vi "Get All Channel Refs.vi"(8 "error in (no error)":errorcluster, 10 "framework configuration in":T1, 11 "VeriStand Data Sharing Framework in":refnum<class "VeriStand DSF.lvclass">) -> (0 "error out":errorcluster, 1 "contiguous?":bool, 2 "all channel offsets":u64[](array[numeric]) format="%.0x", 3 "VeriStand Data Sharing Framework out":refnum<class "VeriStand DSF.lvclass">)   [LabVIEW 2017, in "DSF Engine.lvlib" / "VeriStand DSF.lvclass"]
uses:
  VeriStand DSF.lvclass
  DSF Core.lvlibp/Typedefs/DSF Engine Framework Configuration.ctl
  DSF Core.lvlibp/Typedefs/DSF Engine Plugin Configuration.ctl
  DSF Core.lvlibp/Typedefs/DSF Timing Info.ctl
  DSF Core.lvlibp/Typedefs/DSF Engine Plugin Thread Configuration.ctl
  DSF Core.lvlibp/Typedefs/DSF Settings Info.ctl
  DSF Core.lvlibp/Typedefs/DSF Engine Transfer Group Configuration.ctl
  DSF Core.lvlibp/Typedefs/DSF Direction.ctl
  DSF Core.lvlibp/Typedefs/DSF Engine Transfer Configuration.ctl
  DSF Core.lvlibp/Typedefs/DSF Byte Order.ctl
  DSF Core.lvlibp/Typedefs/DSF Engine Channel Configuration.ctl
  DSF Core.lvlibp/Typedefs/DSF Data Type.ctl
  DSF Core.lvlibp/Typedefs/DSF Timeout Behavior.ctl
  VeriStand DSF.lvclass/VeriStand DSF.ctl
  <vilib>/NI Veristand/Custom Device API/Data Access Type.ctl
  DSF Core.lvlibp/Classes/Configuration/Channel Count (Transfer).vi
  <vilib>/NI Veristand/Custom Device API/Custom Device API.lvlib
  DSF Core.lvlibp
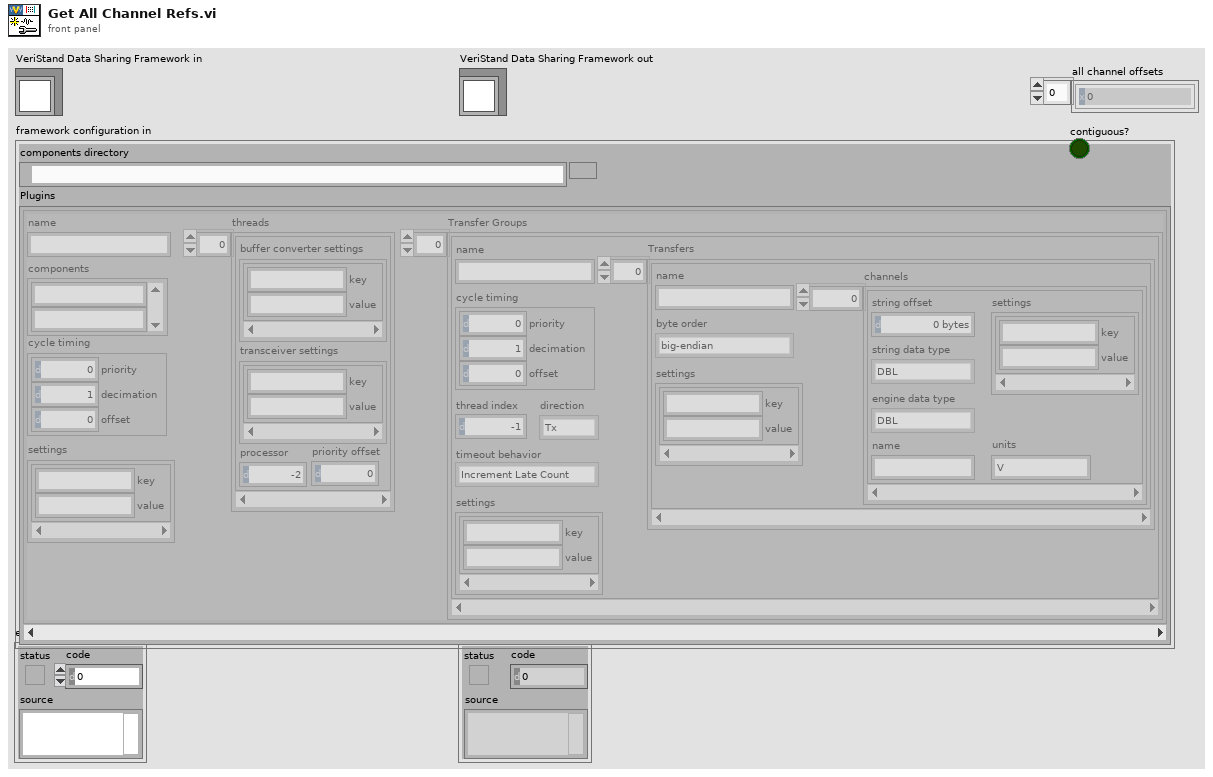
[diagram p1: front panel]
types:
  T1 = typedef "DSF Core.lvlibp/DSF Engine Framework Configuration.ctl" = cluster{"components directory":path, "Plugins":T2[]}
  T2 = typedef "DSF Core.lvlibp/DSF Engine Plugin Configuration.ctl" = cluster{"name":string, "components":string[], "cycle timing":T3, "threads":T4[], "Transfer Groups":T6[], "settings":T5}
  T3 = typedef "DSF Core.lvlibp/DSF Timing Info.ctl" = cluster{"priority":u64, "decimation":u64, "offset":u64}
  T4 = typedef "DSF Core.lvlibp/DSF Engine Plugin Thread Configuration.ctl" = cluster{"buffer converter settings":T5, "transceiver settings":T5, "processor":i32, "priority offset":i16}
  T5 = typedef "DSF Core.lvlibp/DSF Settings Info.ctl" = cluster{"key":string, "value":string}[]
  T6 = typedef "DSF Core.lvlibp/DSF Engine Transfer Group Configuration.ctl" = cluster{"name":string, "direction":T7, "cycle timing":T3, "thread index":i32, "settings":T5, "Transfers":T8[], "timeout behavior":T12}
  T7 = typedef "DSF Core.lvlibp/DSF Direction.ctl" = enum8{"Tx", "Rx"}
  T8 = typedef "DSF Core.lvlibp/DSF Engine Transfer Configuration.ctl" = cluster{"name":string, "byte order":T9, "settings":T5, "channels":T10[]}
  T9 = typedef "DSF Core.lvlibp/DSF Byte Order.ctl" = enum8{"big-endian", "little-endian"}
  T10 = typedef "DSF Core.lvlibp/DSF Engine Channel Configuration.ctl" = cluster{"string offset":u64, "string data type":T11, "engine data type":T11, "name":string, "settings":T5, "units":string}
  T11 = typedef "DSF Core.lvlibp/DSF Data Type.ctl" = enum8{"Bool", "SGL", "DBL", "I8", "I16", "I32", "I64", "U8", "U16", "U32", "U64"}
  T12 = typedef "DSF Core.lvlibp/DSF Timeout Behavior.ctl" = enum8{"Increment Late Count", "Throw Error"}
  T13 = enum16{"open", "replace", "create", "open or create", "replace or create", "replace or create with confirmation"}
  T14 = typedef "Custom Device API.lvlib/Custom Device Item Ref.ctl" = u64
  T15 = typedef "Custom Device API.lvlib/Data Access Type.ctl" = enum16{"Read", "Write"}
  T16 = typedef "Custom Device API.lvlib/Data Reference.ctl" = i32
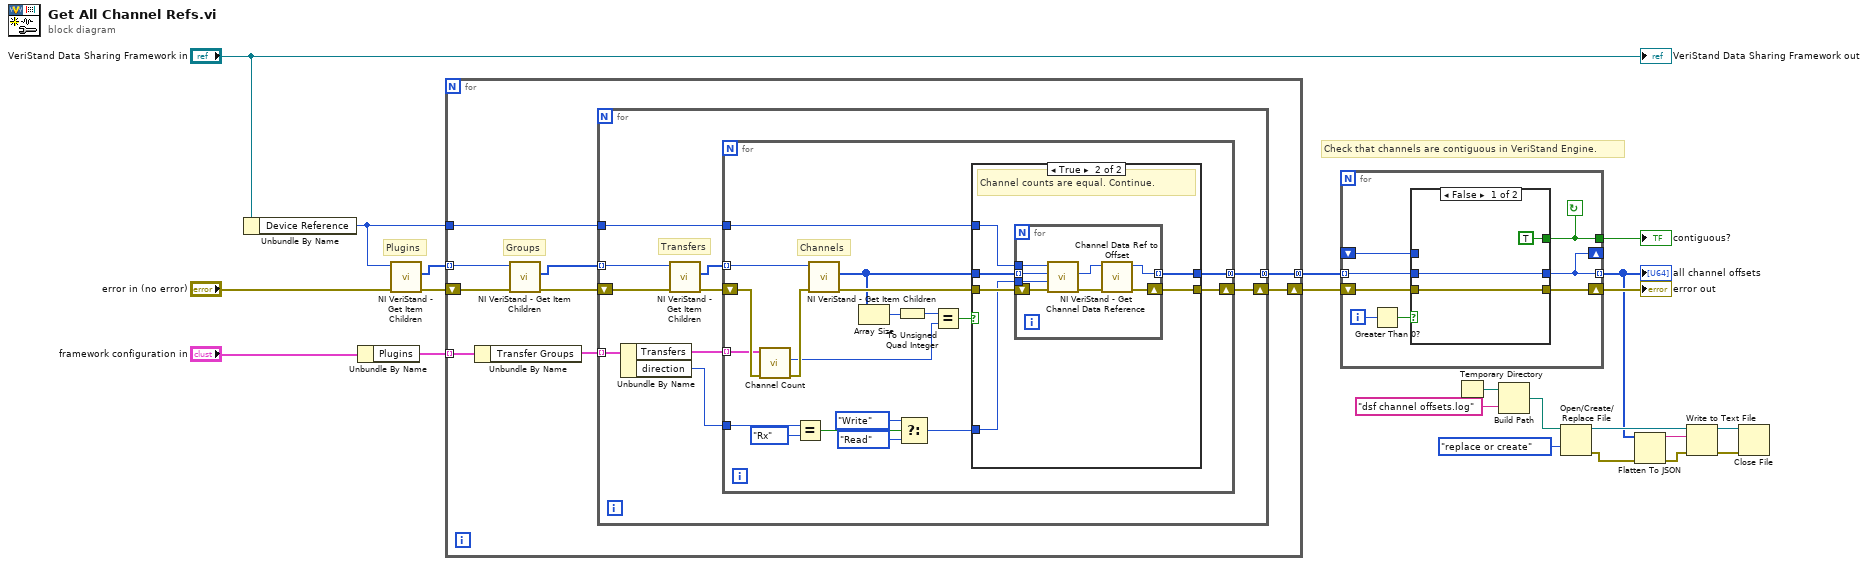
[diagram p0: block diagram]
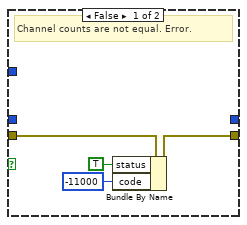
[diagram p2: hidden frame]
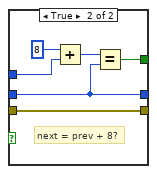
[diagram p3: hidden frame]
diagram:
  # "Check that channels are contiguous in VeriStand Engine."
  # "Plugins"
  n1 = Unbundle By Name("VeriStand Data Sharing Framework in") -> ("Device Reference"=w18:T14)
  n2 = Unbundle By Name("framework configuration in") -> ("Plugins"=w19:T2[])
  n3 = call <vilib>:"NI VeriStand - Get Item Children.vi"("error in (no error)"="error in (no error)", "Item Ref in"=w18) -> ("error out"=w17:errorcluster, "Child Refs"=w20:T14[])  [unwired: 6 in, 2 out]
  n4 = for {
    tunnel: w20 -> [w30] mode=indexing
    tunnel: w19 -> [w31] mode=indexing
    tunnel: w18 -> [w29]
    shift-right: [w27] -> w15
    shift-left: w17 -> [w28]
    tunnel: [w26] -> w14 mode=concatenating
    # "Groups"
    n5 = Unbundle By Name(w31) -> ("Transfer Groups"=w25:T6[])
    n6 = call <vilib>:"NI VeriStand - Get Item Children.vi"("error in (no error)"=w28, "Item Ref in"=w30) -> ("error out"=w23:errorcluster, "Child Refs"=w24:T14[])  [unwired: 6 in, 2 out]
    n7 = for {
      tunnel: w25 -> [w40] mode=indexing
      tunnel: w24 -> [w41] mode=indexing
      tunnel: w29 -> [w39]
      shift-right: [w37] -> w27
      shift-left: w23 -> [w38]
      tunnel: [w36] -> w26 mode=concatenating
      # "Transfers"
      n8 = Unbundle By Name(w40) -> ("Transfers"=w35:T8[], "direction"=w32:T7)
      n9 = call <vilib>:"NI VeriStand - Get Item Children.vi"("error in (no error)"=w38, "Item Ref in"=w41) -> ("error out"=w33:errorcluster, "Child Refs"=w34:T14[])  [unwired: 6 in, 2 out]
      n10 = for {
        tunnel: w35 -> [w44] mode=indexing
        tunnel: w34 -> [w60] mode=indexing
        tunnel: w32 -> [w58]
        tunnel: w39 -> [w51]
        shift-right: [w43] -> w37
        shift-left: w33 -> [w47]
        tunnel: [w42] -> w36 mode=concatenating
        # "Channels"
        n11 = call-poly "Channel Count.vi"("error in (no error)"=w47, "Transfer Configuration in"=w44) -> ("error out"=w46:errorcluster, "total channel count"=w45:u64)  [unwired: 7 in, 1 out]
        n12 = Equal?(x=w58, y=DSF_Direction."Rx") -> (x = y?=w56:bool)
        n13 = call <vilib>:"NI VeriStand - Get Item Children.vi"("error in (no error)"=w46, "Item Ref in"=w60) -> ("error out"=w49:errorcluster, "Child Refs"=w48:T14[])  [unwired: 6 in, 2 out]
        n14 = Array Size(array=w48) -> (size(s)=w59:i32)
        n15 = To Unsigned Quad Integer(1:w59) -> (0:w52:u64)
        n16 = Select(t=Data_Access_Type."Write" ("Access"), s=w56, f=Data_Access_Type."Read") -> (s? t:f=w50:T15)
        n17 = Equal?(x=w52, y=w45) -> (x = y?=w53:bool)
        n18 = case shown="True" w53 {
          tunnel: w48 -> [_ w67]
          tunnel: w51 -> [_ w69]
          tunnel: w50 -> [_ w68]
          tunnel: w49 -> [w64 w70]
          tunnel: [w63 w65] -> w43
          tunnel: [_ w66] -> w42
          frame False {
            # "Channel counts are not equal. Error."
            n19 = Bundle By Name(cluster=w64, "status"=TRUE, "code"=-11000) -> (w63:errorcluster)
          }
          frame True {
            # "Channel counts are equal. Continue."
            n20 = for {
              tunnel: w69 -> [w77]
              tunnel: w68 -> [w76]
              tunnel: w67 -> [w75] mode=indexing
              tunnel: [w71] -> w66 mode=indexing
              shift-right: [w72] -> w65
              shift-left: w70 -> [w78]
              n21 = call <vilib>:"NI VeriStand - Get Channel Data Reference.vi"("error in (no error)"=w78, "Access"=w76, "Channel Ref in"=w75, "Device Ref in"=w77) -> ("error out"=w74:errorcluster, "Channel Data Reference"=w73:T16)  [unwired: 5 in, 1 out]
              n22 = call "Channel Data Ref to Offset.vi"("error in (no error)"=w74, "Channel Data Reference"=w73) -> ("error out"=w72:errorcluster, "channel offset"=w71:u64)  [unwired: 8 in]
            }
          }
        }
      }
    }
  }
  n23 = for {
    tunnel: w14 -> [w84] mode=indexing
    shift-right: [w81] -> w13
    shift-left: w15 -> [w83]
    shift-right: [w79] -> _
    shift-left: _ -> [w82]
    tunnel: [w80] -> w12
    tunnel: [w79] -> w1 mode=indexing
    i -> [w86]
    stop <- w80 continue-if-true
    n24 = Greater Than 0?(x=w86) -> (x > 0?=w85:bool)
    n25 = case shown="False" w85 {
      tunnel: w84 -> [w88 w91]
      tunnel: w83 -> [w89 w90]
      tunnel: w82 -> [_ w95]
      tunnel: [w89 w90] -> w81
      tunnel: [TRUE w92] -> w80
      tunnel: [w88 w91] -> w79
      frame False {
      }
      frame True {
        # "next = prev + 8?"
        n26 = Add(x=u64 8 ("y"), y=w95) -> (x+y=w93:u64)
        n27 = Equal?(x=w93, y=w91) -> (x = y?=w92:bool)
      }
    }
  }
  "error out" <- w13
  "all channel offsets" <- w1
  "contiguous?" <- w12
  n28 = Temporary Directory() -> (w4:path)
  n29 = Build Path(base path=w4, name or relative path="dsf channel offsets.log" ("file path (use dialog)")) -> (appended path=w2:path)
  n30 = Open/Create/Replace File(file path (use dialog)=w2, operation (0:open)=T13."replace or create") -> (refnum out=w7:refnum<file>, error out=w10:errorcluster)  [unwired: 4 in, 1 out]
  n31 = Flatten To JSON(anything=w1, error in (no error)=w10) -> (JSON string=w8:string, 11:w9:errorcluster)  [unwired: 1 in]
  n32 = Write to Text File(file (use dialog)=w7, text=w8, error in=w9) -> (refnum out=w5:refnum<file>, error out=w6:errorcluster)  [unwired: 1 in, 1 out]
  n33 = Close File(refnum=w5, error in=w6) -> ()  [unwired: 2 out]
  "VeriStand Data Sharing Framework out" <- "VeriStand Data Sharing Framework in"
